vi "Ctor.vi"(8 "error in (no error)":errorcluster, 11 "Dashboard Panel in":refnum<class "Dashboard Panel.lvclass">) -> (0 "error out":errorcluster, 3 "Dashboard Panel out":refnum<class "Dashboard Panel.lvclass">)   [LabVIEW 2020, in "SB App.lvlib" / "Dashboard Panel.lvclass"]
uses:
  Dashboard Panel.lvclass
  SquareBattle/Team/Team.lvclass
  Team Status Data.ctl
  SquareBattle/Team Stats.ctl
  SquareBattle/Team State.ctl
  Dashboard Panel.lvclass/Dashboard Panel.ctl
  <vilib>/IlluminatedG/IG OOPanel/OOPanel/Panel/Panel.lvclass
  SquareBattle/SquareBattle.lvlib
  SB App.lvlib
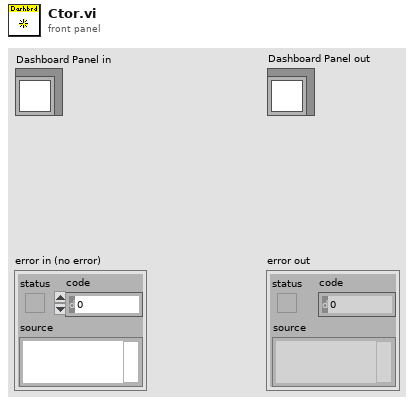
[diagram p1: front panel]
types:
  T1 = typedef "SB App.lvlib/Team Status Data.ctl" = cluster{"Team Stats":T2, "Team State":T3}
  T2 = typedef "SquareBattle.lvlib/Team Stats.ctl" = cluster{"Active":i32, "Generated":i32, "Kills":i32, "Eliminated":i32, "Collided":i32}
  T3 = typedef "SquareBattle.lvlib/Team State.ctl" = enum16{"Active", "Defeated", "Won"}
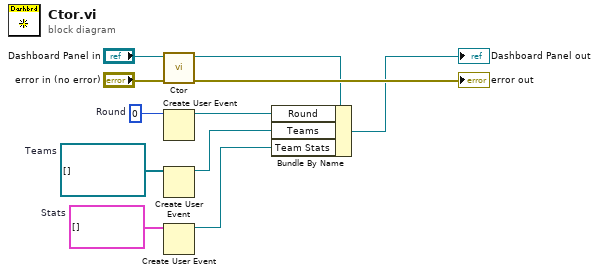
[diagram p0: block diagram]
diagram:
  w2 = T1[] []  # Stats
  w4 = refnum<class "Team.lvclass">[] []  # Teams
  w6 = u32 0  # Round
  n1 = call-parent "Ctor.vi"("error in (no error)"="error in (no error)", "Panel in"="Dashboard Panel in") -> ("error out"=→"error out":errorcluster, "Panel out"=w8:refnum<class "Dashboard Panel.lvclass">)  [unwired: 8 in]
  n2 = Create User Event(user event datatype=w6) -> (user event=w5:refnum<user-event>)  [unwired: 1 in, 1 out]
  n3 = Create User Event(user event datatype=w4) -> (user event=w3:refnum<user-event>)  [unwired: 1 in, 1 out]
  n4 = Create User Event(user event datatype=w2) -> (user event=w1:refnum<user-event>)  [unwired: 1 in, 1 out]
  n5 = Bundle By Name(cluster=w8, "Round"=w5, "Teams"=w3, "Team Stats"=w1) -> (→"Dashboard Panel out":refnum<class "Dashboard Panel.lvclass">)
